vi "Load Module.vi"(8 "error in":errorcluster) -> (0 "error out":errorcluster)   [LabVIEW 2022 SP3, in "Settings.lvlib"]
doc: "Combines Start Module.vi and Synchronize Module Events.vi. Wrapping these allows to programmatically start any module (by use of call by reference) as the module-specific connector panes are hidden away."
uses:
  Settings.lvlib
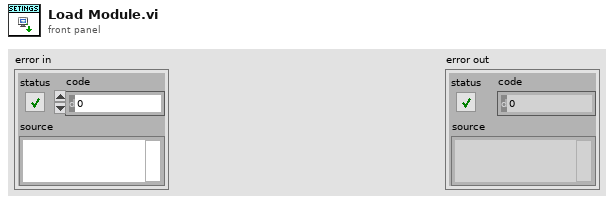
[diagram p1: front panel]
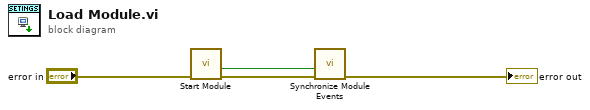
[diagram p0: block diagram]
diagram:
  n1 = call "Start Module.vi"("error in"="error in") -> ("error out"=w3:errorcluster, "Wait for Event Sync?"=w1:bool)  [unwired: 7 in, 2 out]
  n2 = call "Synchronize Module Events.vi"("error in"=w3, "Wait for Event Sync?"=w1) -> ("error out"=→"error out":errorcluster)  [unwired: 9 in]
